vi "Turret_Simulated_Hardware.vi"() -> ()   [LabVIEW 2019]
uses:
  Subsystems/Sensing/Sensor_Values.vi
  Subsystems/Turret/Turret_Globals.vi
panel:
  in  "k_magic":dbl
  out "cowl_acceleration":dbl
  out "true_cowl_velocity":dbl
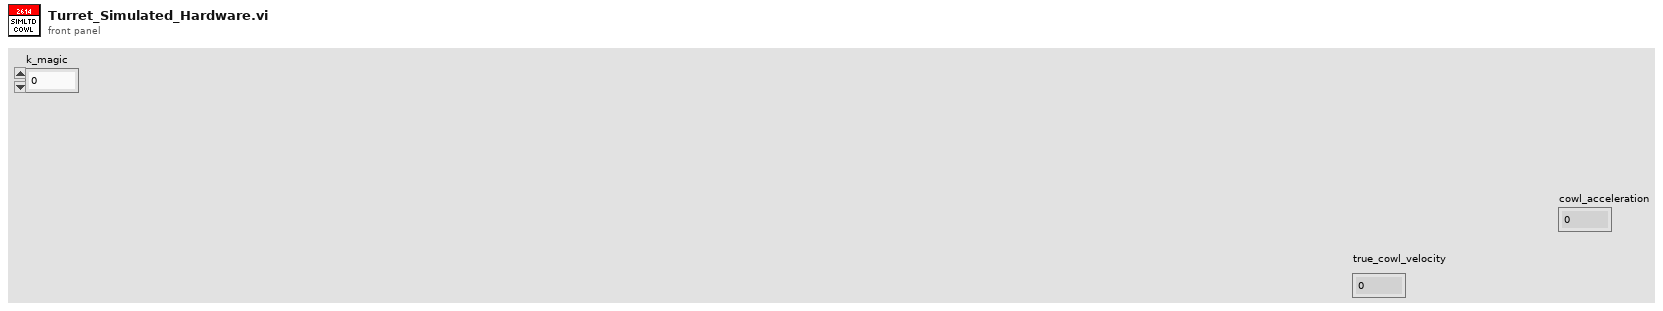
[diagram p1: front panel]
types:
  T1 = typedef "Basic_Motor_Modes.ctl" = enum16{"Percent_Voltage", "Speed_Control", "Position_Control", "Current"}
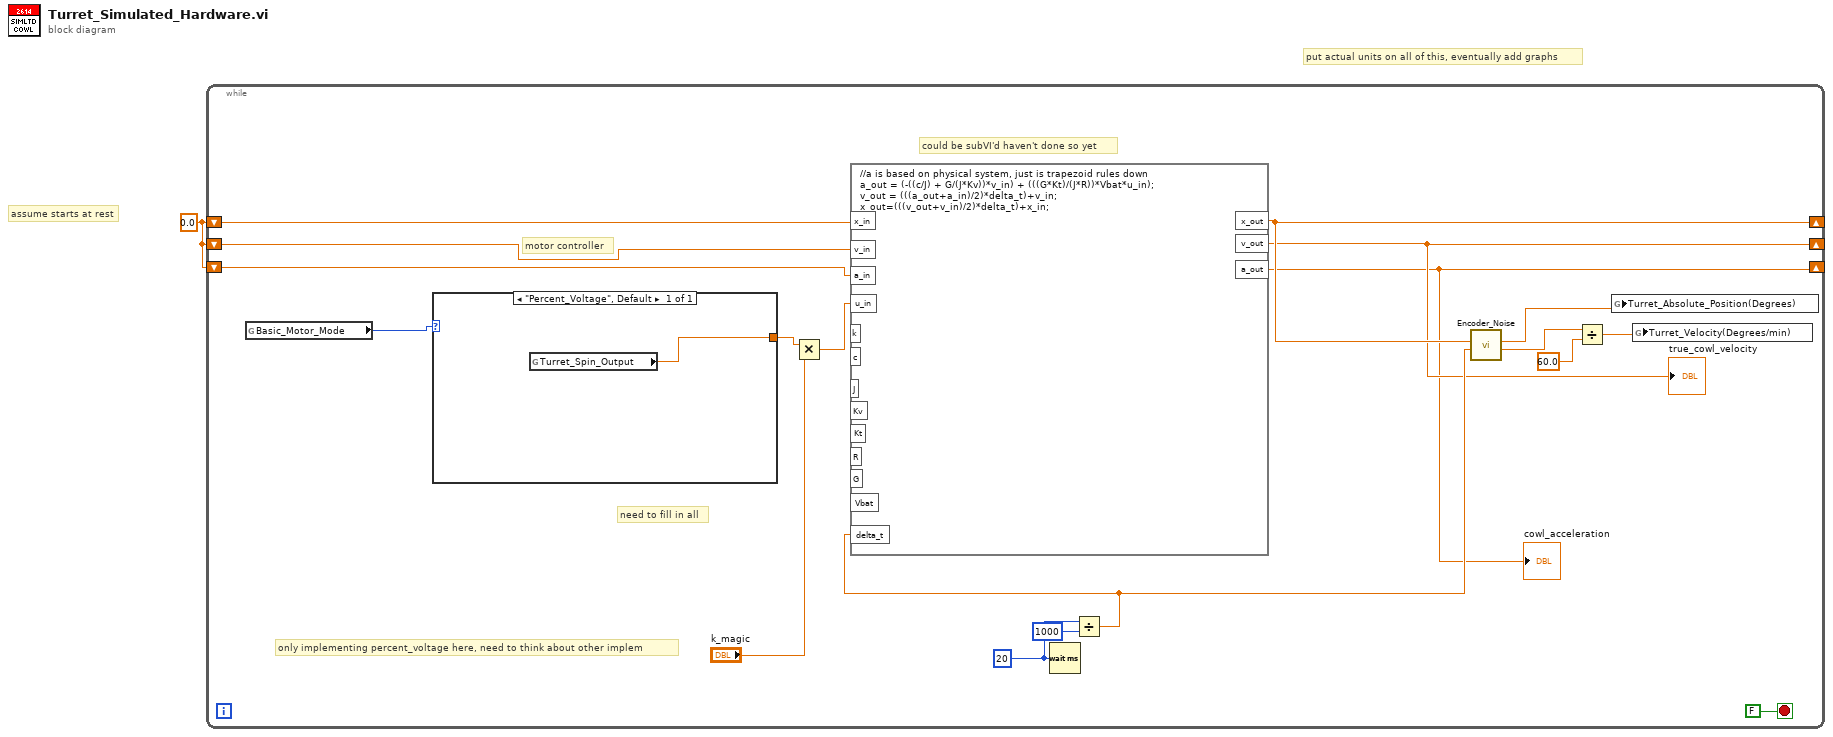
[diagram p0: block diagram]
diagram:
  w1 = 0.0 ("x_out")
  # "assume starts at rest"
  # "put actual units on all of this, eventually add graphs"
  n1 = while {
    shift-right: [w8] -> _
    shift-left: w1 -> [w5]
    shift-right: [w7] -> _
    shift-left: w1 -> [w4]
    shift-right: [w6] -> _
    shift-left: w1 -> [w3]
    stop <- FALSE stop-if-true
    w18 = u32 20 ("milliseconds to wait")
    # "need to fill in all"
    # "could be subVI'd haven't done so yet"
    # "only implementing percent_voltage here, need to think about other implem"
    # "motor controller"
    n2 = global read "Turret_Globals.vi" "Basic_Motor_Mode"() -> (w2:T1)
    n3 = case shown="\"Percent_Voltage\", Default" w2 {
      tunnel: [w20] -> w15
      frame "Percent_Voltage", Default {
        n4 = global read "Turret_Globals.vi" "Turret_Spin_Output"() -> (w20:dbl)
      }
    }
    n5 = Multiply(x=w15, y="k_magic") -> (x*y=w9:dbl)
    n6 = Wait (ms)(milliseconds to wait=w18) -> ()  [unwired: 1 out]
    n7 = Divide(x=w18, y=u32 1000) -> (x/y=w10:dbl)
    n8 = formula code="//a is based on physical system, just is trapezoid rules down\na_out = (-((c/J) + G/(J*Kv))*v_in) + (((G*Kt)/(J*R))*Vbat*u_in);\nv_out = (((a_out+a_in)/2)*delta_t)+v_in;\nx_out=(((v_out+v_in)/2)*delta_t)+x_in;"("x_in"=w5, "v_in"=w4, "a_in"=w3, "u_in"=w9, "delta_t"=w10) -> ("x_out"=w8:dbl, "v_out"=w7:dbl, "a_out"=w6:dbl)  [unwired: 8 in]
    "true_cowl_velocity" <- w7
    "cowl_acceleration" <- w6
    n9 = call "Encoder_Noise.vi"("dt(s)"=w10, "True Position(rotations)"=w8) -> ("Measured Velocity(rotations/sec)"=w14:dbl, "Measured Position(rotations)"=w11:dbl)  [unwired: 8 in]
    n10 = Divide(x=w14, y=60.0) -> (x/y=w12:dbl)
    n11 = global write "Sensor_Values.vi" "Turret_Absolute_Position(Degrees)"(w11) -> ()
    n12 = global write "Sensor_Values.vi" "Turret_Velocity(Degrees/min)"(w12) -> ()
  }
